vi "Update UAV Marker.vi"(7 "Follow?":bool, 8 "Error In":errorcluster, 11 "Selected Aircraft ID in":u8) -> (0 "error out":errorcluster)   [LabVIEW 2014]
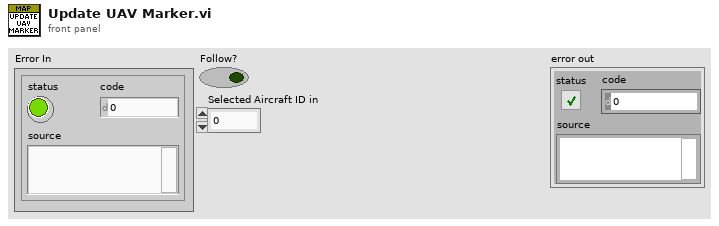
[diagram p1: front panel]
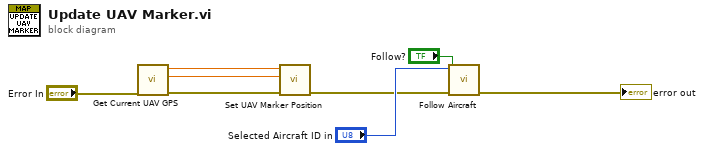
[diagram p0: block diagram]
diagram:
  n1 = call "Get Current UAV GPS.vi"("Error In"="Error In") -> ("Error Out"=w2:errorcluster, "Longitude (degrees)"=w3:dbl, "Latitude (degrees)"=w4:dbl)  [unwired: 8 in]
  n2 = call "Set UAV Marker Position.vi"("error in (no error)"=w2, "lon"=w3, "lat"=w4) -> ("error out"=w1:errorcluster)  [unwired: 8 in]
  n3 = call "Follow Aircraft.vi"("Error In"=w1, "Follow?"="Follow?", "Aircraft ID"="Selected Aircraft ID in") -> ("error out"=→"error out":errorcluster)  [unwired: 8 in]
